vi "Experiment 6.VI"() -> ()   [LabVIEW 2017]
uses:
  <vilib>/DAQmx/write.llb/DAQmx Write (Digital 1D Bool NChan 1Samp 1Line).vi
  <vilib>/DAQmx/read.llb/DAQmx Read (Digital 1D Bool NChan 1Samp 1Line).vi
  <vilib>/DAQmx/read.llb/DAQmx Read (Analog 1D DBL 1Chan NSamp).vi
  <vilib>/DAQmx/create/channels.llb/DAQmx Create Channel (AI-Voltage-Basic).vi
  <vilib>/DAQmx/configure/timing.llb/DAQmx Timing (Sample Clock).vi
  <vilib>/DAQmx/create/channels.llb/DAQmx Create Channel (DI-Digital Input).vi
  <vilib>/DAQmx/create/channels.llb/DAQmx Create Channel (DO-Digital Output).vi
  <vilib>/DAQmx/miscellaneous.llb/DAQmx Fill In Error Info.vi
panel:
  in  "Red LED":bool
  in  "Green LED":bool
  out "Button":bool
  out "Switch":bool
  in  "stop":bool
  out "Potentionmeter":dbl[](graph)
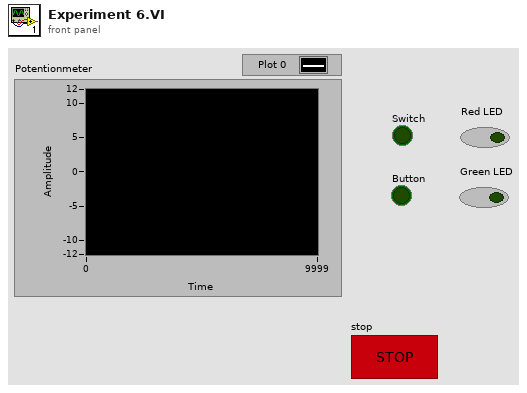
[diagram p1: front panel]
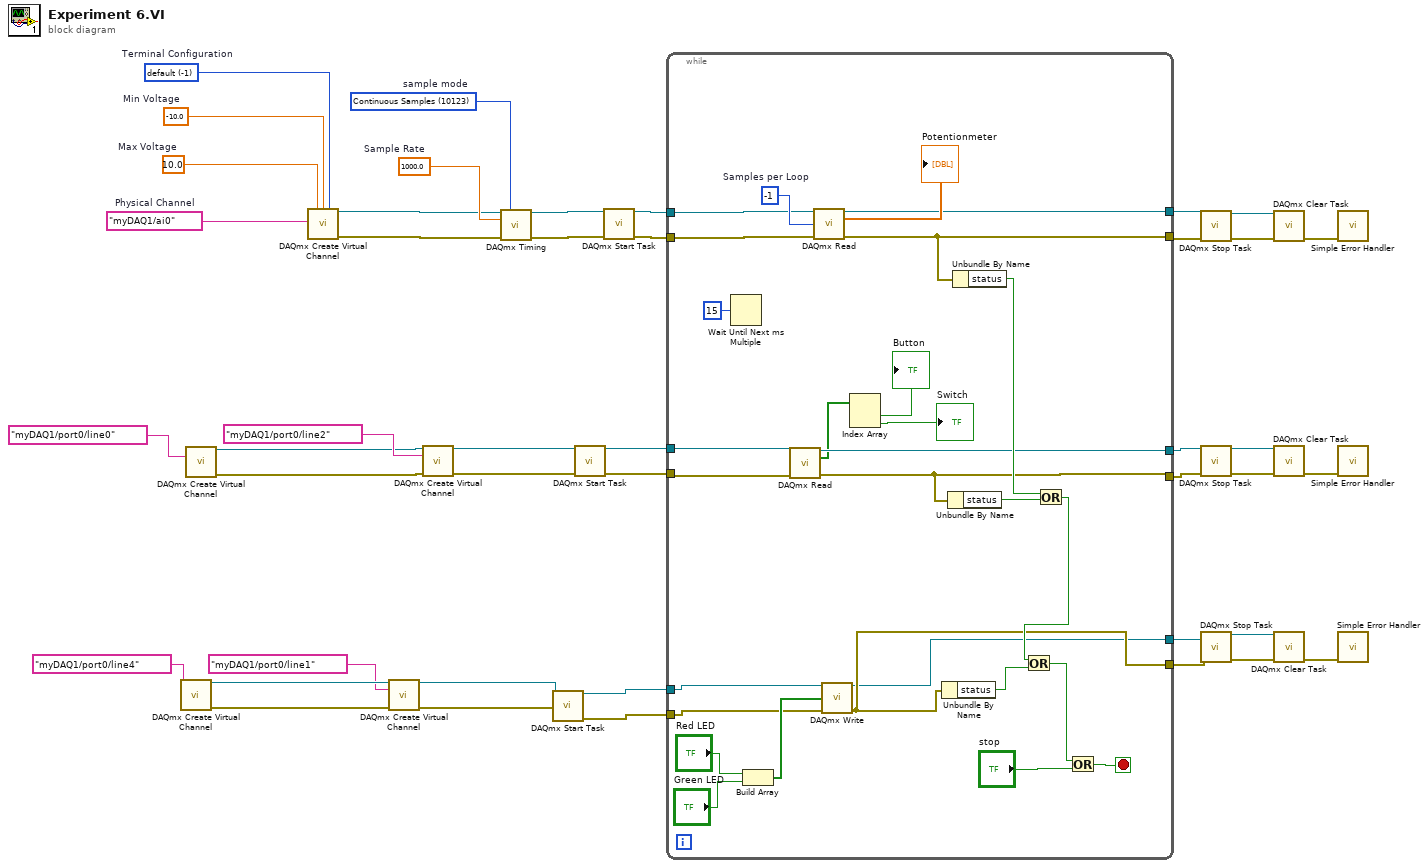
[diagram p0: block diagram]
diagram:
  w38 = 10123 items=["Finite Samples"=10178, "Continuous Samples"=10123, "Hardware Timed Single Point"=12522]  # sample mode
  w39 = 1000.0  # Sample Rate
  w40 = -1 items=["default"=-1, "RSE"=10083, "NRSE"=10078, "Differential"=10106, "Pseudodifferential"=12529]  # Terminal Configuration
  w41 = -10.0  # Min Voltage
  w42 = 10.0  # Max Voltage
  w43 = tag "myDAQ1/ai0"  # Physical Channel
  n1 = call-poly <vilib>:"DAQmx Create Virtual Channel.vi"("lines"=tag "myDAQ1/port0/line4") -> ("task out"=w8:refnum<k21>, "error out"=w7:errorcluster)  [unwired: 13 in]
  n2 = call-poly <vilib>:"DAQmx Create Virtual Channel.vi"("lines"=tag "myDAQ1/port0/line0") -> ("task out"=w16:refnum<k21>, "error out"=w15:errorcluster)  [unwired: 13 in]
  n3 = call-poly <vilib>:"DAQmx Create Virtual Channel.vi"("maximum value"=w42, "minimum value"=w41, "input terminal configuration"=w40, "physical channels"=w43) -> ("task out"=w36:refnum<k21>, "error out"=w37:errorcluster)  [unwired: 10 in]
  n4 = call-poly <vilib>:"DAQmx Create Virtual Channel.vi"("task in"=w8, "lines"=tag "myDAQ1/port0/line1", "error in"=w7) -> ("task out"=w6:refnum<k21>, "error out"=w5:errorcluster)  [unwired: 11 in]
  n5 = call-poly <vilib>:"DAQmx Create Virtual Channel.vi"("task in"=w16, "lines"=tag "myDAQ1/port0/line2", "error in"=w15) -> ("task out"=w25:refnum<k21>, "error out"=w24:errorcluster)  [unwired: 11 in]
  n6 = call-poly <vilib>:"DAQmx Timing.vi"("task/channels in"=w36, "sample mode"=w38, "rate"=w39, "error in"=w37) -> ("task out"=w35:refnum<k21>, "error out"=w34:errorcluster)  [unwired: 10 in]
  n7 = call <vilib>:"DAQmx Start Task.vi"("task/channels in"=w6, "error in"=w5) -> ("task out"=w4:refnum<k21>, "error out"=w3:errorcluster)  [unwired: 12 in]
  n8 = call <vilib>:"DAQmx Start Task.vi"("task/channels in"=w25, "error in"=w24) -> ("task out"=w23:refnum<k21>, "error out"=w22:errorcluster)  [unwired: 12 in]
  n9 = call <vilib>:"DAQmx Start Task.vi"("task/channels in"=w35, "error in"=w34) -> ("task out"=w33:refnum<k21>, "error out"=w32:errorcluster)  [unwired: 12 in]
  n10 = while {
    tunnel: w33 -> [w68]
    tunnel: w32 -> [w69]
    tunnel: [w64] -> w29
    tunnel: [w63] -> w28
    tunnel: w23 -> [w61]
    tunnel: w22 -> [w60]
    tunnel: [w59] -> w18
    tunnel: [w57] -> w17
    tunnel: [w50] -> w12
    tunnel: [w49] -> w13
    tunnel: w4 -> [w46]
    tunnel: w3 -> [w47]
    stop <- w66 stop-if-true
    w70 = -1  # Samples per Loop
    n11 = Wait Until Next ms Multiple(millisecond multiple=u32 15) -> ()  [unwired: 1 out]
    n12 = Build Array("Red LED", "Green LED") -> (w48:bool[])
    n13 = call-poly <vilib>:"DAQmx Read.vi"("task/channels in"=w61, "error in"=w60) -> ("task out"=w57:refnum<k21>, "data"=w56:bool[], "error out"=w59:errorcluster)  [unwired: 11 in]
    n14 = call-poly <vilib>:"DAQmx Read.vi"("task/channels in"=w68, "number of samples per channel"=w70, "error in"=w69) -> ("task out"=w63:refnum<k21>, "data"=→"Potentionmeter":dbl[], "error out"=w64:errorcluster)  [unwired: 10 in]
    n15 = call-poly <vilib>:"DAQmx Write.vi"("task/channels in"=w46, "data"=w48, "error in"=w47) -> ("task out"=w49:refnum<k21>, "error out"=w50:errorcluster)  [unwired: 10 in, 1 out]
    n16 = Index Array(array=w56) -> (element #1=→"Button":bool, element #2=→"Switch":bool)  [unwired: 2 in]
    n17 = Unbundle By Name(w50) -> ("status"=w51:bool)
    n18 = Unbundle By Name(w59) -> ("status"=w58:bool)
    n19 = Unbundle By Name(w64) -> ("status"=w62:bool)
    n20 = Or(x=w62, y=w58) -> (x .or. y?=w53:bool)
    n21 = Or(x=w53, y=w51) -> (x .or. y?=w52:bool)
    n22 = Or(x=w52, y="stop") -> (x .or. y?=w66:bool)
  }
  n23 = call <vilib>:"DAQmx Stop Task.vi"("task/channels in"=w28, "error in"=w29) -> ("task out"=w31:refnum<k21>, "error out"=w30:errorcluster)  [unwired: 12 in]
  n24 = call <vilib>:"DAQmx Stop Task.vi"("task/channels in"=w17, "error in"=w18) -> ("task out"=w21:refnum<k21>, "error out"=w20:errorcluster)  [unwired: 12 in]
  n25 = call <vilib>:"DAQmx Stop Task.vi"("task/channels in"=w13, "error in"=w12) -> ("task out"=w11:refnum<k21>, "error out"=w10:errorcluster)  [unwired: 12 in]
  n26 = call <vilib>:"DAQmx Clear Task.vi"("task in"=w31, "error in"=w30) -> ("error out"=w27:errorcluster)  [unwired: 13 in]
  n27 = call <vilib>:"DAQmx Clear Task.vi"("task in"=w21, "error in"=w20) -> ("error out"=w19:errorcluster)  [unwired: 13 in]
  n28 = call <vilib>:"DAQmx Clear Task.vi"("task in"=w11, "error in"=w10) -> ("error out"=w9:errorcluster)  [unwired: 13 in]
  n29 = call <vilib>:"Simple Error Handler.vi"("error in (no error)"=w27) -> ()  [unwired: 4 in, 5 out]
  n30 = call <vilib>:"Simple Error Handler.vi"("error in (no error)"=w19) -> ()  [unwired: 4 in, 5 out]
  n31 = call <vilib>:"Simple Error Handler.vi"("error in (no error)"=w9) -> ()  [unwired: 4 in, 5 out]
